vi "obstacles.vi"() -> (7 "appended array":cluster{"x1":dbl[], "y1":dbl[]}[](array[cluster]))   [LabVIEW 2017]
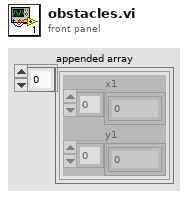
[diagram p1: front panel]
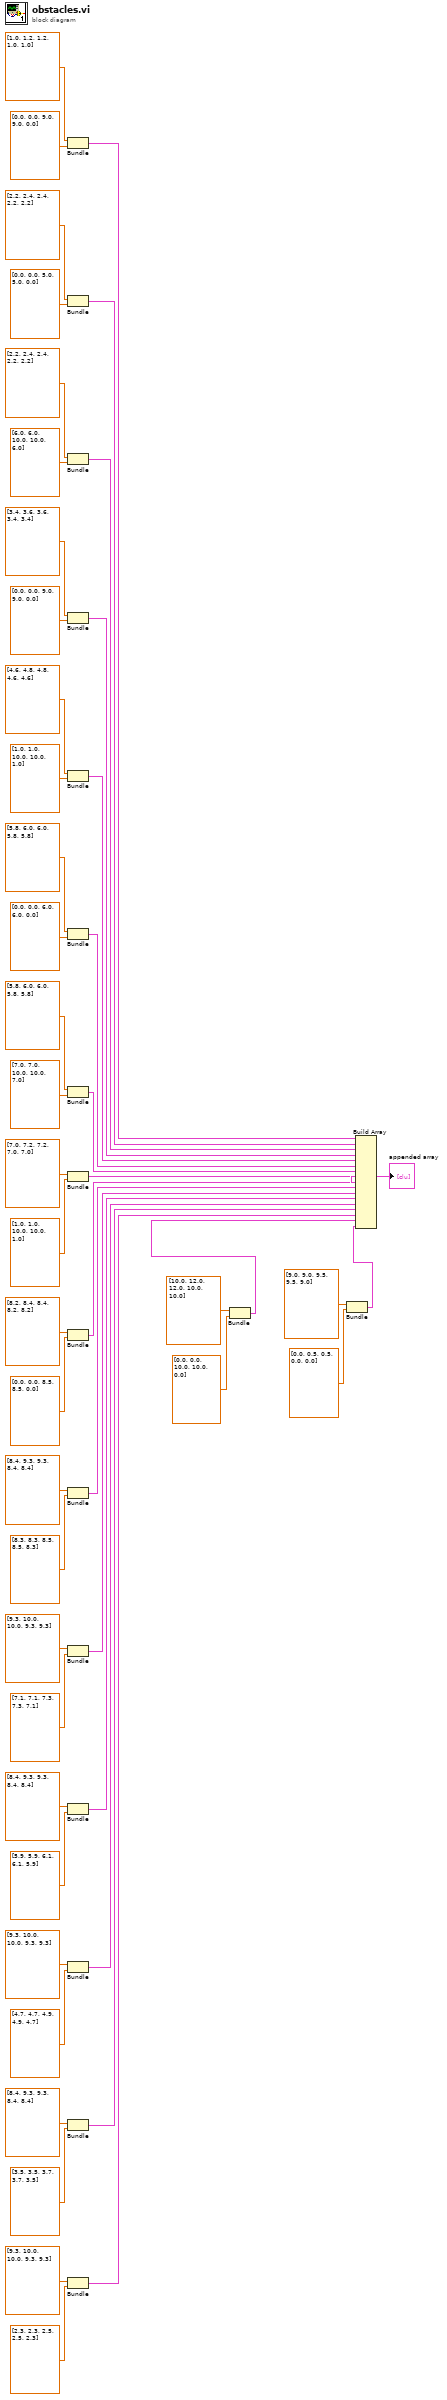
[diagram p0: block diagram]
diagram:
  n1 = Bundle("x1"=dbl[] [1.0, 1.2, 1.2, 1.0, 1.0], "y1"=dbl[] [0.0, 0.0, 9.0, 9.0, 0.0]) -> (w48:cluster{"x1":dbl[], "y1":dbl[]})  [unwired: 1 in]
  n2 = Bundle("x1"=dbl[] [2.2, 2.4, 2.4, 2.2, 2.2], "y1"=dbl[] [0.0, 0.0, 5.0, 5.0, 0.0]) -> (w47:cluster{"x1":dbl[], "y1":dbl[]})  [unwired: 1 in]
  n3 = Bundle("x1"=dbl[] [2.2, 2.4, 2.4, 2.2, 2.2], "y1"=dbl[] [6.0, 6.0, 10.0, 10.0, 6.0]) -> (w37:cluster{"x1":dbl[], "y1":dbl[]})  [unwired: 1 in]
  n4 = Bundle("x1"=dbl[] [3.4, 3.6, 3.6, 3.4, 3.4], "y1"=dbl[] [0.0, 0.0, 9.0, 9.0, 0.0]) -> (w36:cluster{"x1":dbl[], "y1":dbl[]})  [unwired: 1 in]
  n5 = Bundle("x1"=dbl[] [4.6, 4.8, 4.8, 4.6, 4.6], "y1"=dbl[] [1.0, 1.0, 10.0, 10.0, 1.0]) -> (w35:cluster{"x1":dbl[], "y1":dbl[]})  [unwired: 1 in]
  n6 = Bundle("x1"=dbl[] [5.8, 6.0, 6.0, 5.8, 5.8], "y1"=dbl[] [0.0, 0.0, 6.0, 6.0, 0.0]) -> (w34:cluster{"x1":dbl[], "y1":dbl[]})  [unwired: 1 in]
  n7 = Bundle("x1"=dbl[] [5.8, 6.0, 6.0, 5.8, 5.8], "y1"=dbl[] [7.0, 7.0, 10.0, 10.0, 7.0]) -> (w29:cluster{"x1":dbl[], "y1":dbl[]})  [unwired: 1 in]
  n8 = Bundle("x1"=dbl[] [7.0, 7.2, 7.2, 7.0, 7.0], "y1"=dbl[] [1.0, 1.0, 10.0, 10.0, 1.0]) -> (w28:cluster{"x1":dbl[], "y1":dbl[]})  [unwired: 1 in]
  n9 = Bundle("x1"=dbl[] [8.2, 8.4, 8.4, 8.2, 8.2], "y1"=dbl[] [0.0, 0.0, 8.5, 8.5, 0.0]) -> (w19:cluster{"x1":dbl[], "y1":dbl[]})  [unwired: 1 in]
  n10 = Bundle("x1"=dbl[] [8.4, 9.3, 9.3, 8.4, 8.4], "y1"=dbl[] [8.3, 8.3, 8.5, 8.5, 8.3]) -> (w18:cluster{"x1":dbl[], "y1":dbl[]})  [unwired: 1 in]
  n11 = Bundle("x1"=dbl[] [9.3, 10.0, 10.0, 9.3, 9.3], "y1"=dbl[] [7.1, 7.1, 7.3, 7.3, 7.1]) -> (w17:cluster{"x1":dbl[], "y1":dbl[]})  [unwired: 1 in]
  n12 = Bundle("x1"=dbl[] [8.4, 9.3, 9.3, 8.4, 8.4], "y1"=dbl[] [5.9, 5.9, 6.1, 6.1, 5.9]) -> (w16:cluster{"x1":dbl[], "y1":dbl[]})  [unwired: 1 in]
  n13 = Bundle("x1"=dbl[] [9.3, 10.0, 10.0, 9.3, 9.3], "y1"=dbl[] [4.7, 4.7, 4.9, 4.9, 4.7]) -> (w9:cluster{"x1":dbl[], "y1":dbl[]})  [unwired: 1 in]
  n14 = Bundle("x1"=dbl[] [8.4, 9.3, 9.3, 8.4, 8.4], "y1"=dbl[] [3.5, 3.5, 3.7, 3.7, 3.5]) -> (w8:cluster{"x1":dbl[], "y1":dbl[]})  [unwired: 1 in]
  n15 = Bundle("x1"=dbl[] [9.3, 10.0, 10.0, 9.3, 9.3], "y1"=dbl[] [2.3, 2.3, 2.5, 2.5, 2.3]) -> (w7:cluster{"x1":dbl[], "y1":dbl[]})  [unwired: 1 in]
  n16 = Bundle("x1"=dbl[] [10.0, 12.0, 12.0, 10.0, 10.0], "y1"=dbl[] [0.0, 0.0, 10.0, 10.0, 0.0]) -> (w4:cluster{"x1":dbl[], "y1":dbl[]})  [unwired: 1 in]
  n17 = Bundle("x1"=dbl[] [9.0, 9.0, 9.5, 9.5, 9.0], "y1"=dbl[] [0.0, 0.5, 0.5, 0.0, 0.0]) -> (w1:cluster{"x1":dbl[], "y1":dbl[]})  [unwired: 1 in]
  n18 = Build Array(w48, w47, w37, w36, w35, w34, w29, w28, w19, w18, w17, w16, w9, w8, w7, w4, w1) -> (→"appended array":cluster{"x1":dbl[], "y1":dbl[]}[])
